vi "Read Measurement 2 Channels.vi"(6 "Measurement Type (0: Phase)":i32(ring) items=["Phase", "Delay", "DelayRR", "DelayRF", "DelayFR", "DelayFF"], 8 "error in (no error)":errorcluster, 9 "Channel 2 (2: Channel 2)":i32(ring)=2 items=["Channel 1"=1, "Channel 2"=2, "Channel 3"=3, "Channel 4"=4], 10 "Channel 1 (1: Channel 1)":i32(ring)=1 items=["Channel 1"=1, "Channel 2"=2, "Channel 3"=3, "Channel 4"=4], 11 "TDS 2000 in":refnum<class "TDS 2000.lvclass">) -> (0 "error out":errorcluster, 1 "Units":string, 2 "Measurement":dbl, 3 "TDS 2000 out":refnum<class "TDS 2000.lvclass">)   [LabVIEW 2020, in "Oscilloscope.lvlib" / "TDS 2000.lvclass"]
uses:
  TDS 2000.lvclass
  C:/Users/ronad/Osciloscopio/Osciloscopio DQMH/Libraries/Oscilloscope/Clases/Osciloscopio/Osciloscopio.lvclass
  Osciloscopio/Osciloscopio.lvclass/Osciloscopio.ctl
  Osciloscopio/Read COM.vi
  Osciloscopio/Write COM.vi
  <instrlib>/Tektronix TDS 200 1000 2000 Series/Tektronix TDS 200 1000 2000 Series.lvlib
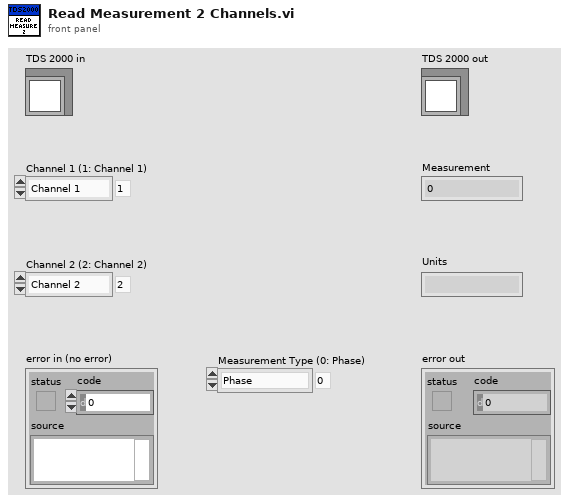
[diagram p1: front panel]
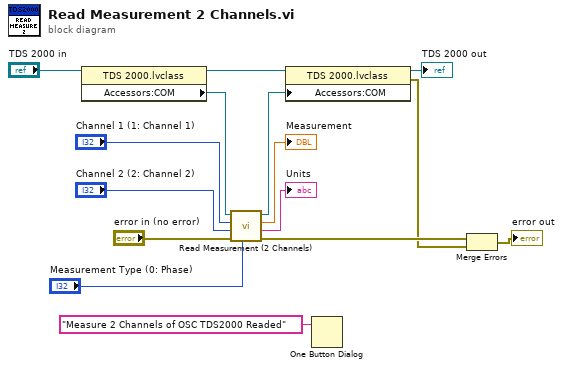
[diagram p0: block diagram]
diagram:
  n1 = property class="TDS 2000.lvclass"(reference="TDS 2000 in") -> (reference out=w13:refnum<class "TDS 2000.lvclass">, "Accessors:COM"=w14:refnum<visa-resource-name>)  [unwired: 1 in, 1 out]
  n2 = call <instrlib>:"Read Measurement (2 Channels).vi"("Measurement Type (0: Phase)"="Measurement Type (0: Phase)", "error in (no error)"="error in (no error)", "Channel 2 (2: Channel 2)"="Channel 2 (2: Channel 2)", "Channel 1 (1: Channel 1)"="Channel 1 (1: Channel 1)", "VISA resource name"=w14) -> ("error out"=w6:errorcluster, "Units"=→"Units":string, "Measurement"=→"Measurement":dbl, "VISA resource name out"=w12:refnum<visa-resource-name>)  [unwired: 3 in]
  n3 = property class="TDS 2000.lvclass"(reference=w13, "Accessors:COM"=w12) -> (reference out=→"TDS 2000 out":refnum<class "TDS 2000.lvclass">, error out=w2:errorcluster)  [unwired: 1 in]
  n4 = One Button Dialog(message="Measure 2 Channels of OSC TDS2000 Readed") -> ()  [unwired: 1 in, 1 out]
  n5 = Merge Errors(w6, w2) -> (→"error out":errorcluster)
